vi "PH_Countdown-Counter.ProcPeriodic.vi"(0 "i ref in":refnum<vi>, 3 "ms timeout (100)":i32=100, 5 "error in (no error)":errorcluster) -> (14 "i ref out":refnum<vi>, 17 "timed out":bool, 19 "error out":errorcluster)   [LabVIEW 2014, in "PH_Countdown-Counter.lvlib"]
doc: "This method serves to periodically do things like reading values from the HW. Methods that should be executed periodically should be called from THIS methode. Add code here."
uses:
  PH_Countdown-Counter.lvlib
  PH_Classes/PH_Sound/PH_Sound.lvlib
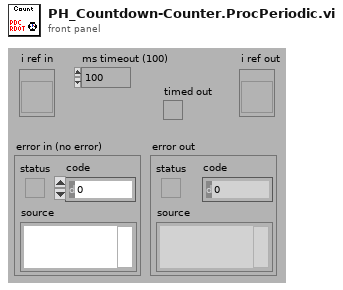
[diagram p1: front panel]
types:
  T1 = typedef "PH_Countdown-Counter.lvlib/PH_Countdown-Counter.i attribute.ctl" = cluster{"Machine Time":cluster{"Tag":string, "Wating Time [s]":dbl, "not linked?":bool}[], "Last Shot":cluster{"Tag":string, "Shot Time [s]":timestamp, "not linked?":bool}[], "Time since last Shot?":bool, "Calculation":cluster{"Time between Shots [s]":dbl, "Ref Remaining Time":refnum<vi>, "Service ID":i32, "over?":bool, "Ref Time between Shots":refnum<vi>, "Ref Set Mode":refnum<vi>}, "Sound?":bool, "Reminder":cluster{"# 1":cluster{"Pretime [s]":dbl, "Aktive?":bool, "Over?":bool}, "# 2":cluster{"Pretime [s]":dbl, "Aktive?":bool, "Over?":bool}}, "MainAmp only":cluster{"State":bool, "GUI Ref":refnum<vi>}}
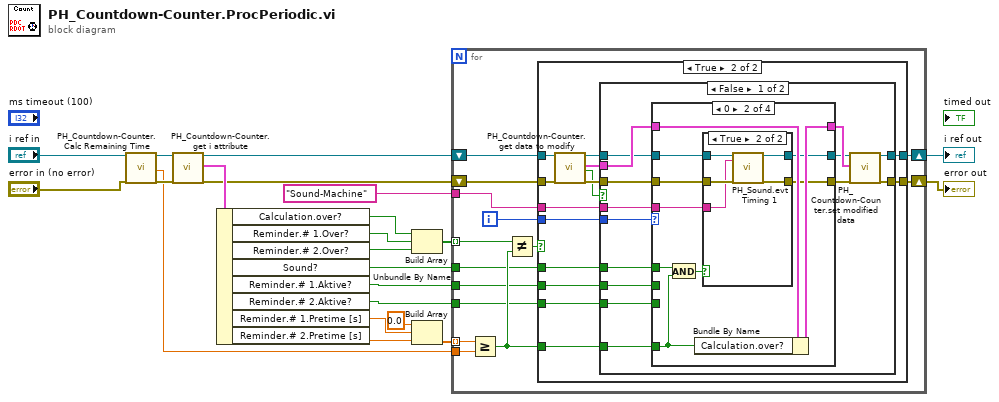
[diagram p0: block diagram]
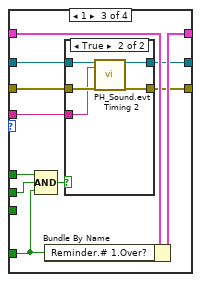
[diagram p5: hidden frame]
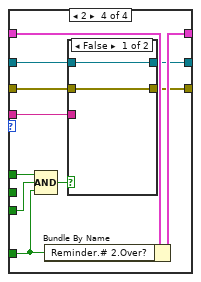
[diagram p7: hidden frame]
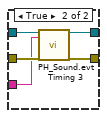
[diagram p8: hidden frame]
diagram:
  n1 = call "PH_Countdown-Counter.Calc Remaining Time.vi"("i ref in"="i ref in", "error in"="error in (no error)") -> ("i ref out"=w21:refnum<vi>, "remaining Time [s]"=w19:dbl, "error out"=w22:errorcluster)  [unwired: 15 in]
  n2 = call "PH_Countdown-Counter.get i attribute.vi"("i ref in"=w21, "error in (no error)"=w22) -> ("i ref out"=w9:refnum<vi>, "i attribute"=w20:T1, "error out"=w10:errorcluster)  [unwired: 15 in]
  n3 = Unbundle By Name(w20) -> ("Calculation.over?"=w15:bool, "Reminder.# 1.Over?"=w14:bool, "Reminder.# 2.Over?"=w13:bool, "Sound?"=w6:bool, "Reminder.# 1.Aktive?"=w5:bool, "Reminder.# 2.Aktive?"=w4:bool, "Reminder.# 1.Pretime [s]"=w18:dbl, "Reminder.# 2.Pretime [s]"=w17:dbl)
  n4 = Build Array(w15, w14, w13) -> (w11:bool[])
  n5 = Build Array(0.0 ("element"), w18, w17) -> (w12:dbl[])
  n6 = for {
    tunnel: w19 -> [w36]
    tunnel: w12 -> [w35] mode=indexing
    tunnel: w11 -> [w28] mode=indexing
    shift-right: [w32] -> w8
    shift-left: w9 -> [w33]
    shift-right: [w31] -> w7
    shift-left: w10 -> [w34]
    tunnel: w6 -> [w26]
    tunnel: w5 -> [w25]
    tunnel: w4 -> [w24]
    tunnel: "Sound-Machine" ("Instance") -> [w23]
    i -> [w27]
    n7 = Greater Or Equal?(x=w35, y=w36) -> (x >= y?=w30:bool)
    n8 = Not Equal?(x=w28, y=w30) -> (x != y?=w29:bool)
    n9 = case shown="True" w29 {
      tunnel: w34 -> [w37 w48]
      tunnel: w33 -> [w38 w47]
      tunnel: [w38 w46] -> w32
      tunnel: [w37 w45] -> w31
      tunnel: w30 -> [_ w44]
      tunnel: w27 -> [_ w43]
      tunnel: w26 -> [_ w42]
      tunnel: w25 -> [_ w41]
      tunnel: w24 -> [_ w40]
      tunnel: w23 -> [_ w39]
      frame False {
      }
      frame True {
        n10 = call "PH_Countdown-Counter.get data to modify.vi"("i ref in"=w47, "error in (no error)"=w48) -> ("i ref out"=w51:refnum<vi>, "i attribute"=w49:T1, "timed out"=w50:bool, "error out"=w52:errorcluster)  [unwired: 14 in]
        n11 = case shown="False" w50 {
          tunnel: w52 -> [w57 w123]
          tunnel: [w66 w123] -> w45
          tunnel: w51 -> [w55 w124]
          tunnel: [w65 w124] -> w46
          tunnel: w49 -> [w64 _]
          tunnel: w44 -> [w62 _]
          tunnel: w43 -> [w61 _]
          tunnel: w42 -> [w60 _]
          tunnel: w41 -> [w59 _]
          tunnel: w40 -> [w58 _]
          tunnel: w39 -> [w53 _]
          frame False {
            n12 = case shown="0" w61 {
              tunnel: w64 -> [w69 w79 w97 w115]
              tunnel: [w69 w78 w96 w114] -> w63
              tunnel: w62 -> [_ w76 w95 w113]
              tunnel: w60 -> [_ w77 w87 w106]
              tunnel: w59 -> [_ _ w88 _]
              tunnel: w58 -> [_ _ _ w105]
              tunnel: w57 -> [w67 w75 w94 w112]
              tunnel: [w67 w74 w93 w111] -> w56
              tunnel: w55 -> [w68 w73 w92 w110]
              tunnel: [w68 w72 w91 w109] -> w54
              tunnel: w53 -> [_ w71 w90 w108]
              frame Default {
              }
              frame 0 {
                n13 = And(x=w77, y=w76) -> (x .and. y?=w70:bool)
                n14 = Bundle By Name(cluster=w79, "Calculation.over?"=w76) -> (w78:T1)
                n15 = case shown="True" w70 {
                  tunnel: w75 -> [w80 w86]
                  tunnel: [w80 w85] -> w74
                  tunnel: w73 -> [w81 w84]
                  tunnel: [w81 w83] -> w72
                  tunnel: w71 -> [_ w82]
                  frame False {
                  }
                  frame True {
                    n16 = call "PH_Sound.evt Timing 1.vi"("i ref in"=w84, "Instance"=w82, "error in (no error)"=w86) -> ("i ref out"=w83:refnum<vi>, "error out"=w85:errorcluster)  [unwired: 15 in]
                  }
                }
              }
              frame 1 {
                n17 = Compound Arithmetic op=AND(w87, w88, w95) -> (w89:bool)
                n18 = Bundle By Name(cluster=w97, "Reminder.# 1.Over?"=w95) -> (w96:T1)
                n19 = case shown="True" w89 {
                  tunnel: w94 -> [w98 w104]
                  tunnel: [w98 w103] -> w93
                  tunnel: w92 -> [w99 w102]
                  tunnel: [w99 w101] -> w91
                  tunnel: w90 -> [_ w100]
                  frame False {
                  }
                  frame True {
                    n20 = call "PH_Sound.evt Timing 2.vi"("i ref in"=w102, "Instance"=w100, "error in (no error)"=w104) -> ("i ref out"=w101:refnum<vi>, "error out"=w103:errorcluster)  [unwired: 15 in]
                  }
                }
              }
              frame 2 {
                n21 = Compound Arithmetic op=AND(w106, w105, w113) -> (w107:bool)
                n22 = Bundle By Name(cluster=w115, "Reminder.# 2.Over?"=w113) -> (w114:T1)
                n23 = case shown="False" w107 {
                  tunnel: w112 -> [w116 w122]
                  tunnel: [w116 w121] -> w111
                  tunnel: w110 -> [w117 w120]
                  tunnel: [w117 w119] -> w109
                  tunnel: w108 -> [_ w118]
                  frame False {
                  }
                  frame True {
                    n24 = call "PH_Sound.evt Timing 3.vi"("i ref in"=w120, "Instance"=w118, "error in (no error)"=w122) -> ("i ref out"=w119:refnum<vi>, "error out"=w121:errorcluster)  [unwired: 15 in]
                  }
                }
              }
            }
            n25 = call "PH_Countdown-Counter.set modified data.vi"("i ref in"=w54, "i attribute"=w63, "error in (no error)"=w56) -> ("i ref out"=w65:refnum<vi>, "error out"=w66:errorcluster)  [unwired: 15 in]
          }
          frame True {
          }
        }
      }
    }
  }
  "error out" <- w7
  "i ref out" <- w8
